vi "G_Posiciones_Finales.vi"() -> ()   [LabVIEW 2020]
panel:
  in  "Posiciones finales":T1={"Desmenuzadora F (x)"=110.0, "Desmenuzadora F (y)"=180.0, "Aspa F (x) "=135.0, "Aspa F (y)"=231.0, "Masa elvador F (x)"=636.0, "Masa elevador F (y)"=24.0, "Galletas Molde F (x)"=1063.0, "Galletas Molde F (y)"=169.0, "Galletas Horno F (x) "=181.0, "Galletas Horno F (y) "=361.0, "Galletas Enfria F (x)"=1073.0, "Galletas Enfria F (y) "=558.0}
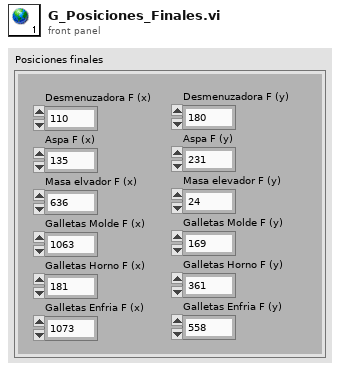
[diagram p1: front panel]
types:
  T1 = cluster{"Desmenuzadora F (x)":dbl, "Desmenuzadora F (y)":dbl, "Aspa F (x) ":dbl, "Aspa F (y)":dbl, "Masa elvador F (x)":dbl, "Masa elevador F (y)":dbl, "Galletas Molde F (x)":dbl, "Galletas Molde F (y)":dbl, "Galletas Horno F (x) ":dbl, "Galletas Horno F (y) ":dbl, "Galletas Enfria F (x)":dbl, "Galletas Enfria F (y) ":dbl}
diagram:
